vi "OperateStringTime.vi"(7 "caculation":enum16{"add", "minus"}(ring), 10 "Second":dbl, 11 "StringTime":string) -> (3 "StringTime":string)   [LabVIEW 2018]
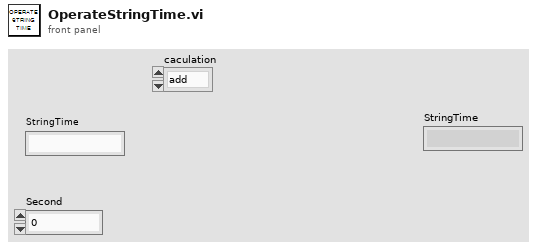
[diagram p1: front panel]
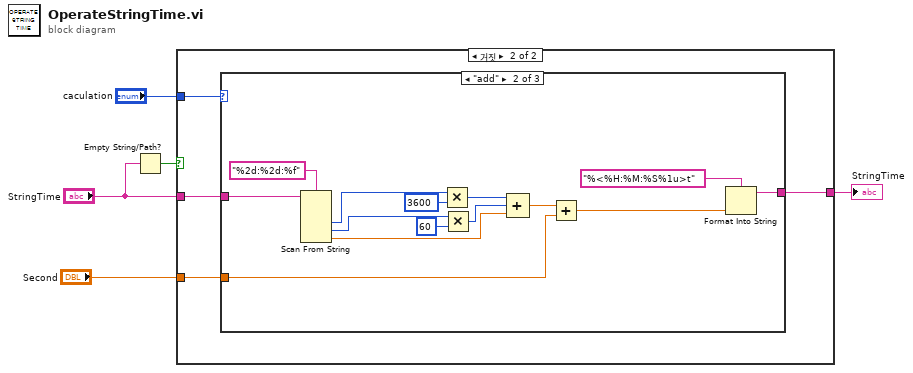
[diagram p0: block diagram]
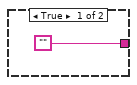
[diagram p2: hidden frame]
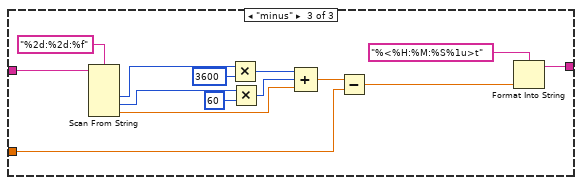
[diagram p4: hidden frame]
diagram:
  n1 = Empty String/Path?(string/path="StringTime") -> (empty?=w5:bool)
  n2 = case shown="거짓" w5 {
    tunnel: "StringTime" -> [_ w10]
    tunnel: "Second" -> [_ w9]
    tunnel: ["" w8] -> w2
    tunnel: "caculation" -> [_ w7]
    frame True {
    }
    frame False {
      n3 = case shown="\"add\"" w7 {
        tunnel: w10 -> [w11 w17 w31]
        tunnel: w9 -> [_ w15 w29]
        tunnel: [w11 w12 w26] -> w8
        frame Default {
        }
        frame "add" {
          n4 = Scan From String(format string="%2d:%2d:%f" ("포맷 문자열"), input string=w17) -> (output 1=w24:i32, output 2=w22:i32, output 3=w18:dbl)  [unwired: 5 in, 3 out]
          n5 = Multiply(x=w24, y=3600) -> (x*y=w20:i32)
          n6 = Multiply(x=w22, y=60) -> (x*y=w19:i32)
          n7 = Compound Arithmetic op=ADD(w20, w19, w18) -> (w16:dbl)
          n8 = Add(x=w16, y=w15) -> (x+y=w14:dbl)
          n9 = Format Into String(format string="%<%H:%M:%S%1u>t", w14) -> (resulting string=w12:string)  [unwired: 2 in, 1 out]
        }
        frame "minus" {
          n10 = Scan From String(format string="%2d:%2d:%f" ("포맷 문자열"), input string=w31) -> (output 1=w38:i32, output 2=w36:i32, output 3=w32:dbl)  [unwired: 5 in, 3 out]
          n11 = Multiply(x=w38, y=3600) -> (x*y=w34:i32)
          n12 = Multiply(x=w36, y=60) -> (x*y=w33:i32)
          n13 = Compound Arithmetic op=ADD(w34, w33, w32) -> (w30:dbl)
          n14 = Subtract(x=w30, y=w29) -> (x-y=w28:dbl)
          n15 = Format Into String(format string="%<%H:%M:%S%1u>t", w28) -> (resulting string=w26:string)  [unwired: 2 in, 1 out]
        }
      }
    }
  }
  "StringTime" <- w2
